vi "p01 Counter.vi"() -> ()   [LabVIEW 2025]
uses:
  <vilib>/rvi/Emulation/niFpgaGetClockAttributes.vi
  <vilib>/rvi/Emulation/niFpgaSctlEmulationGetInTimedLoop.vi
  <vilib>/rvi/Emulation/niFpgaEmulationReportErrorSimple.vi
  <vilib>/rvi/Emulation/niFpgaCriticalErrorInLSC.vi
panel:
  in  "Reset":bool
  out "Count":u32
  in  "Up":bool
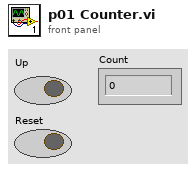
[diagram p1: front panel]
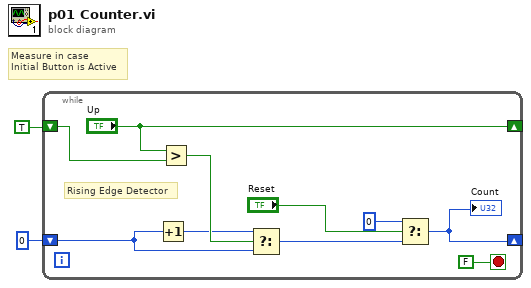
[diagram p0: block diagram]
diagram:
  # "Measure in case \nInitial Button is Active"
  n1 = while {
    shift-right: ["Up"] -> _
    shift-left: TRUE ("Up") -> [w10]
    shift-right: [w5] -> _
    shift-left: u32 0 -> [w7]
    stop <- FALSE stop-if-true
    # "Rising Edge Detector"
    n2 = Increment(x=w7) -> (x+1=w8:u32)
    n3 = Greater?(x="Up", y=w10) -> (0:w9:bool)
    n4 = Select(t=w8, s=w9, f=w7) -> (s? t:f=w4:u32)
    n5 = Select(t=u32 0, s="Reset", f=w4) -> (s? t:f=w5:u32)
    "Count" <- w5
  }
